vi "CodeKeithley.vi"(8 "Program":string, 11 "SweepInfo":T1={"Current Range"=1e-10, "Source Measure Unit Channel (0: Channel A)"=0, "Waveform"={"t0"=timestamp(0 s since 1904-01-01), "dt"=1.0, "Y"=[]}, "VISA resource name"="", "CodeText"=""}) -> (0 "error out":errorcluster)   [LabVIEW 2020]
uses:
  Keithley 2600 Series/Keithley 2600 Series.lvlib
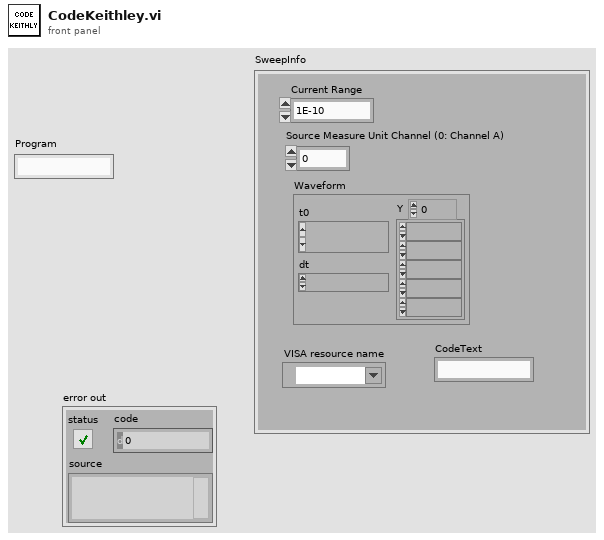
[diagram p1: front panel]
types:
  T1 = cluster{"Current Range":dbl, "Source Measure Unit Channel (0: Channel A)":i32, "Waveform":waveform(dbl), "VISA resource name":refnum<visa-resource-name>, "CodeText":string}
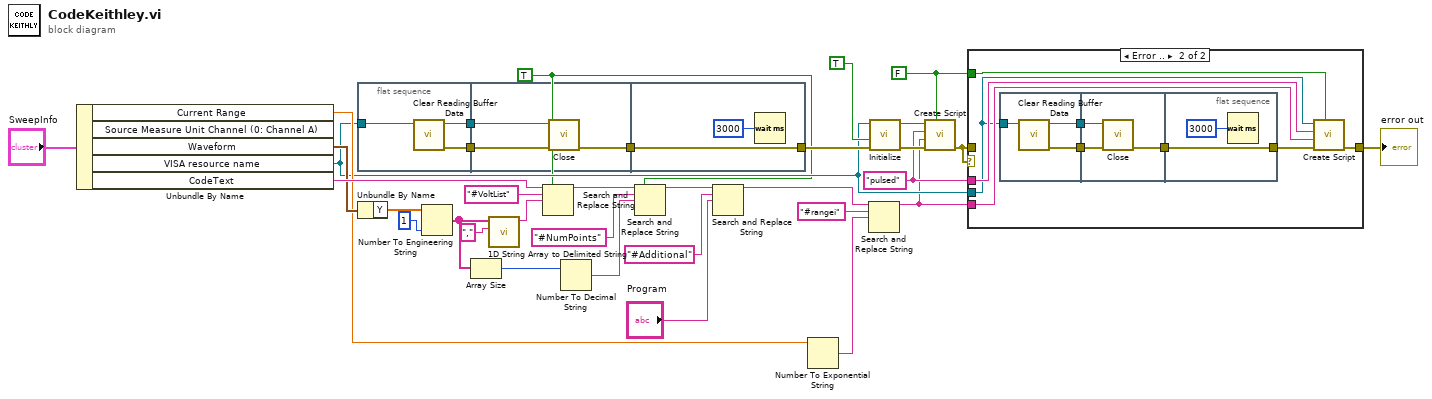
[diagram p0: block diagram]
diagram:
  w1 = TRUE ("replace all? (F)")
  w4 = "pulsed" ("Script Variable")
  w2 = FALSE ("Auto Run (F: Disable)")
  n1 = Unbundle By Name("SweepInfo") -> ("Current Range"=w16:dbl, "Waveform"=w18:waveform(dbl), "VISA resource name"=w7:refnum<visa-resource-name>, "CodeText"=w19:string)  [unwired: 1 out]
  n2 = flat-sequence {
    tunnel: w7 -> [w37]
    tunnel: [w36] -> w15
    tunnel: [w35] -> w14
    tunnel: w15 -> [w40]
    tunnel: w14 -> [w39]
    tunnel: [w38] -> w13
    tunnel: [w41] -> w12
    tunnel: w13 -> [w41]
    frame #0 {
      n3 = call "Clear Reading Buffer Data.vi"("VISA resource name"=w37) -> ("error out"=w36:errorcluster, "VISA resource name out"=w35:refnum<visa-resource-name>)  [unwired: 9 in]
    }
    frame #1 {
      n4 = call "Close.vi"("error in (no error)"=w40, "VISA resource name"=w39) -> ("error out"=w38:errorcluster)  [unwired: 9 in]
    }
    frame #2 {
      n5 = Wait (ms)(milliseconds to wait=u32 3000) -> ()  [unwired: 1 out]
    }
  }
  n6 = Unbundle By Name(w18) -> ("Y"=w30:dbl[])
  n7 = Number To Engineering String(2:i16 1 ("precision (6)"), 4:w30) -> (0:w23:string[])  [unwired: 2 in]
  n8 = Array Size(array=w23) -> (size(s)=w22:i32)
  n9 = call <vilib>:"1D String Array to Delimited String.vi"("delimiter"=",", "string array"=w23) -> ("delimited string"=w25:string)  [unwired: 9 in]
  n10 = Search and Replace String(replace all?=w1, input string=w19, search string="#VoltList", replace string=w25) -> (result string=w24:string)  [unwired: 4 in, 3 out]
  n11 = Number To Decimal String(number=w22) -> (decimal integer string=w21:string)  [unwired: 1 in]
  n12 = Search and Replace String(replace all?=w1, input string=w24, search string="#NumPoints", replace string=w21) -> (result string=w10:string)  [unwired: 4 in, 3 out]
  n13 = Search and Replace String(input string=w10, search string="#Additional", replace string="Program") -> (result string=w11:string)  [unwired: 5 in, 3 out]
  n14 = Number To Exponential String(number=w16) -> (E-format string=w20:string)  [unwired: 3 in]
  n15 = Search and Replace String(input string=w11, search string="#rangei", replace string=w20) -> (result string=w3:string)  [unwired: 5 in, 3 out]
  n16 = call "Initialize.vi"("error in (no error)"=w12, "Reset (True)"=TRUE, "VISA resource name"=w7) -> ("error out"=w33:errorcluster, "VISA resource name out"=w32:refnum<visa-resource-name>)  [unwired: 7 in]
  n17 = call "Create Script.vi"("Auto Run (F: Disable)"=w2, "error in (no error)"=w33, "Source Code"=w3, "Script Variable"=w4, "VISA resource name"=w32) -> ("error out"=w5:errorcluster)  [unwired: 5 in, 1 out]
  n18 = case shown="Error .." w5 {
    tunnel: w7 -> [_ w44]
    tunnel: [w43 w45] -> w6
    tunnel: w5 -> [w43 _]
    tunnel: w4 -> [_ w49]
    tunnel: w3 -> [_ w48]
    tunnel: w2 -> [_ w47]
    frame No Error {
    }
    frame Error {
      n19 = flat-sequence {
        tunnel: [w55] -> w52
        tunnel: [w54] -> w51
        tunnel: w44 -> [w53]
        tunnel: w52 -> [w58]
        tunnel: w51 -> [w57]
        tunnel: [w56] -> w50
        tunnel: [w59] -> w46
        tunnel: w50 -> [w59]
        frame #0 {
          n20 = call "Clear Reading Buffer Data.vi"("VISA resource name"=w53) -> ("error out"=w55:errorcluster, "VISA resource name out"=w54:refnum<visa-resource-name>)  [unwired: 9 in]
        }
        frame #1 {
          n21 = call "Close.vi"("error in (no error)"=w58, "VISA resource name"=w57) -> ("error out"=w56:errorcluster)  [unwired: 9 in]
        }
        frame #2 {
          n22 = Wait (ms)(milliseconds to wait=u32 3000) -> ()  [unwired: 1 out]
        }
      }
      n23 = call "Create Script.vi"("Auto Run (F: Disable)"=w47, "error in (no error)"=w46, "Source Code"=w48, "Script Variable"=w49, "VISA resource name"=w44) -> ("error out"=w45:errorcluster)  [unwired: 5 in, 1 out]
    }
  }
  "error out" <- w6
